vi "Teleop.vi"(10 "Match Info":T1={"Autonomous Elapsed Seconds"=0.0, "TeleOp Elapsed Seconds"=84.436, "Disabled Elapsed Seconds"=0.0, "Visited Autonomous"=FALSE, "Visited TeleOp"=TRUE, "Visited Disabled"=FALSE, "Autonomous Settings"={"Autonomous Style"=enum."Independent", "VI Refnum"=refnum}}, 11 "Call Context":T2=enum."Execute") -> ()   [LabVIEW 2012]
doc: "This VI is called for each TeleOp packet received from the DS where the robot is not disabled. It is often used to read from the joysticks and update I/O or to update setpoints for timed control loops. It should complete and return within 20 milliseconds or it may miss DS packets."
uses:
  <vilib>/Rock Robotics/WPI/DriverStation/WPI_DriverStationDerivedRobotMode.ctl
  <vilib>/Rock Robotics/WPI/DriverStation/WPI_DriverStationMatch Info.ctl
  Controls/Jaguar Control Modes.ctl
  Controls/Robot Orientation.ctl
  Robot Global Data.vi
  Globals/Jaguar Control Mode.vi
  Globals/Autonomous Tipping.vi
  Autonomous/Autonomous Shooting.vi
  Globals/Are We Calibrating Steering.vi
  Globals/DriveSystemMode.vi
  Globals/Max Robot Speed.vi
  Globals/Jaguar Commands.vi
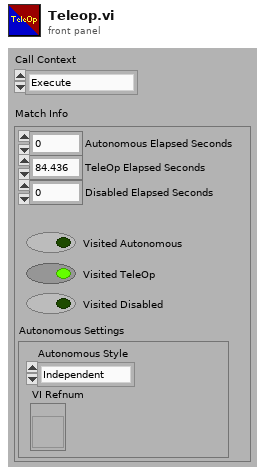
[diagram p1: front panel]
types:
  T1 = typedef "WPI_DriverStationMatch Info.ctl" = cluster{"Autonomous Elapsed Seconds":dbl, "TeleOp Elapsed Seconds":dbl, "Disabled Elapsed Seconds":dbl, "Visited Autonomous":bool, "Visited TeleOp":bool, "Visited Disabled":bool, "Autonomous Settings":cluster{"Autonomous Style":enum16{"Iterative", "Independent"}, "VI Refnum":refnum<vi>}}
  T2 = typedef "WPI_DriverStationDerivedRobotMode.ctl" = enum16{"Init", "Execute", "Stop"}
  T3 = typedef "Jaguar Control Modes.ctl" = enum16{"Speed", "Position"}
  T4 = typedef "Drive System Mode.ctl" = enum16{"Normal", "Crab", "Shoot"}
  T5 = typedef "Robot Orientation.ctl" = enum16{"Landscape", "Portrait"}
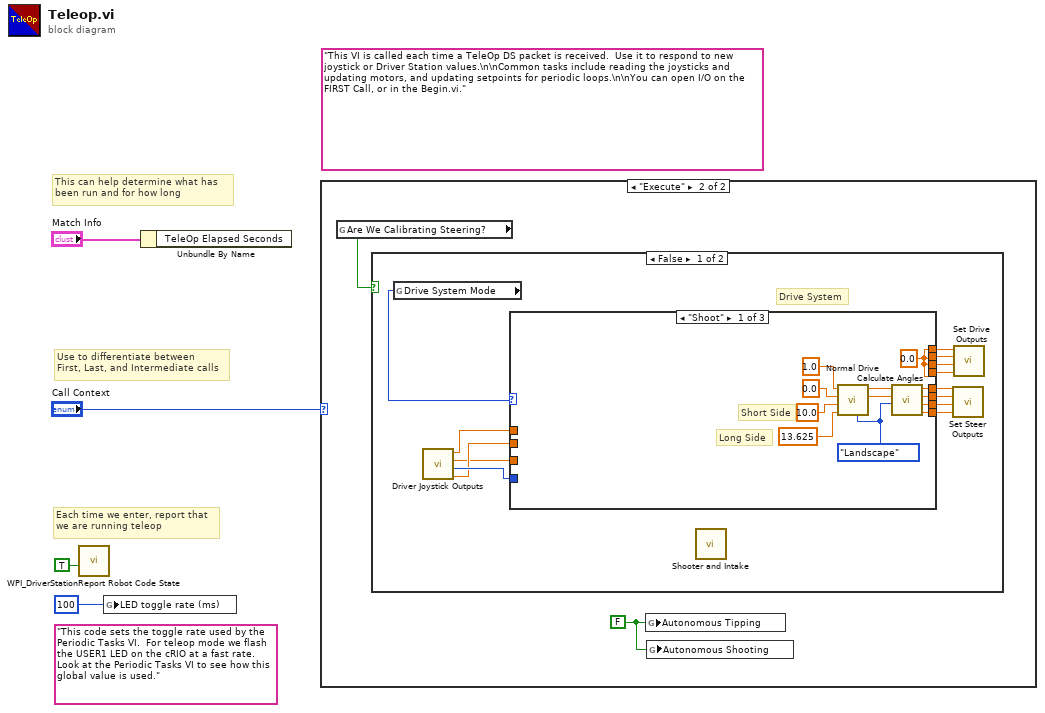
[diagram p0: block diagram]
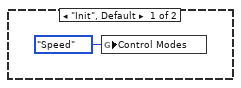
[diagram p2: hidden frame]
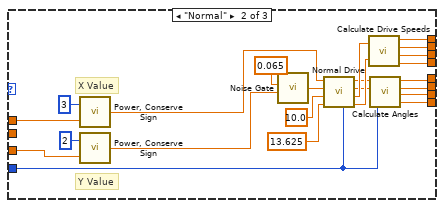
[diagram p3: hidden frame]
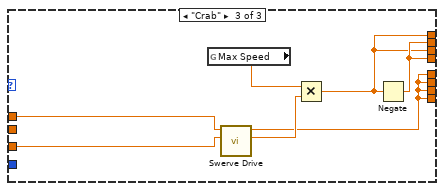
[diagram p4: hidden frame]
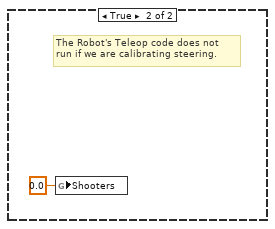
[diagram p5: hidden frame]
diagram:
  (unwired) "This code sets the toggle rate used by the Periodic Tasks VI.  For teleop mode we flash the USER1 LED on the cRIO at a fast rate.  Look at the Periodic Tasks VI to see how this global value is used."
  (unwired) "This VI is called each time a TeleOp DS packet is received.  Use it to respond to new joystick or Driver Station values.\n\nCommon tasks include reading the joysticks and updating motors, and updating setpoints for periodic loops.\n\nYou can open I/O on the FIRST Call, or in the Begin.vi."
  # "Each time we enter, report that\nwe are running teleop"
  # "Use to differentiate between\nFirst, Last, and Intermediate calls"
  # "This can help determine what has\nbeen run and for how long"
  n1 = call <vilib>:"WPI_DriverStationReport Robot Code State.vi"("TeleOp"=TRUE ("Autonomous")) -> ()  [unwired: 10 in, 1 out]
  n2 = global write "Robot Global Data.vi" "LED toggle rate (ms)"(u32 100 ("LED ms toggle rate")) -> ()
  n3 = Unbundle By Name("Match Info") -> ()  [unwired: 1 out]
  n4 = case shown="\"Execute\"" "Call Context" {
    frame "Init", Default {
      n5 = global write "Jaguar Control Mode.vi" "Control Modes"(Jaguar_Control_Modes."Speed" ("Mode")) -> ()
    }
    frame "Execute" {
      w6 = FALSE ("Autonomous Tipping")
      n6 = global read "Are We Calibrating Steering.vi" "Are We Calibrating Steering?"() -> (w7:bool)
      n7 = case shown="False" w7 {
        frame False {
          # "Drive System"
          n8 = global read "DriveSystemMode.vi" "Drive System Mode"() -> (w20:T4)
          n9 = call "Driver Joystick Outputs.vi"() -> ("Joy X"=w8:dbl, "Joy Y"=w9:dbl, "Robot Orientation"=w11:T5, "Joy Twist"=w10:dbl)  [unwired: 3 in]
          n10 = case shown="\"Shoot\"" w20 {
            tunnel: [w28 w47 w60] -> w15
            tunnel: w10 -> [_ _ _]
            tunnel: w9 -> [_ w35 w56]
            tunnel: [w21 w42 w58] -> w19
            tunnel: [w21 w41 w59] -> w18
            tunnel: [w21 w40 w58] -> w17
            tunnel: [w21 w39 w59] -> w16
            tunnel: [w27 w46 w60] -> w14
            tunnel: [w26 w45 w60] -> w13
            tunnel: [w25 w44 w60] -> w12
            tunnel: w11 -> [_ w43 _]
            tunnel: w8 -> [_ w34 w57]
            frame "Shoot" {
              w21 = 0.0 ("Front Left Speed")
              w22 = Robot_Orientation."Landscape" ("Robot Orientation")
              # "Long Side"
              # "Short Side"
              n11 = call "Normal Drive.vi"("Joy X"=1.0, "Joy Y"=0.0, "Short Radius (Inches)"=10.0 ("Vertical Radius (Inches)"), "Long Radius (Inches)"=13.625 ("Lateral Radius (Inches)"), "Robot Orientation"=w22) -> ("Front Left Angle Out"=w24:dbl, "Front Right Angle Out"=w23:dbl)  [unwired: 1 in, 2 out]
              n12 = call "Calculate Angles.vi"("Robot Orientation"=w22, "Right Angle In"=w23, "Left Angle In"=w24) -> ("Rear Right Steer Out"=w25:dbl, "Rear Left Pot Out"=w26:dbl, "Front Right Pot Out"=w27:dbl, "Front Left Pot Out"=w28:dbl)  [unwired: 1 in]
            }
            frame "Normal" {
              # "Y Value"
              # "X Value"
              n13 = call "Power, Conserve Sign.vi"("Input"=w34, "Power"=3) -> ("Output"=w38:dbl)  [unwired: 1 in]
              n14 = call "Power, Conserve Sign.vi"("Input"=w35, "Power"=2) -> ("Output"=w36:dbl)  [unwired: 1 in]
              n15 = call "Noise Gate.vi"("Gate Value"=0.065, "Value In"=w36) -> ("Value Out"=w52:dbl)  [unwired: 5 in]
              n16 = call "Normal Drive.vi"("Joy X"=w38, "Joy Y"=w52, "Short Radius (Inches)"=10.0 ("Vertical Radius (Inches)"), "Long Radius (Inches)"=13.625 ("Lateral Radius (Inches)"), "Robot Orientation"=w43) -> ("Front Left Angle Out"=w49:dbl, "Front Right Angle Out"=w48:dbl, "Left Speed Out"=w51:dbl, "Right Speed Out"=w50:dbl)  [unwired: 1 in]
              n17 = call "Calculate Drive Speeds.vi"("Left Speed In"=w51, "Right Speed In"=w50) -> ("Front Left Speed"=w42:dbl, "Front Right Speed"=w41:dbl, "Rear Left Speed"=w40:dbl, "Rear Right Speed"=w39:dbl)  [unwired: 2 in]
              n18 = call "Calculate Angles.vi"("Robot Orientation"=w43, "Right Angle In"=w48, "Left Angle In"=w49) -> ("Rear Right Steer Out"=w44:dbl, "Rear Left Pot Out"=w45:dbl, "Front Right Pot Out"=w46:dbl, "Front Left Pot Out"=w47:dbl)  [unwired: 1 in]
            }
            frame "Crab" {
              n19 = global read "Max Robot Speed.vi" "Max Speed"() -> (w62:dbl)
              n20 = call "Swerve Drive.vi"("Joy Y"=w56, "Joy X"=w57) -> ("Speed"=w61:dbl, "Wheel Angle"=w60:dbl)  [unwired: 8 in]
              n21 = Multiply(x=w62, y=w61) -> (x*y=w58:dbl)
              n22 = Negate(x=w58) -> (-x=w59:dbl)
            }
          }
          n23 = call "Shooter and Intake.vi"() -> ()  [unwired: 1 in]
          n24 = call "Set Steer Outputs.vi"("Rear Right"=w12, "Rear Left"=w13, "Front Right"=w14, "Front Left"=w15) -> ()  [unwired: 8 in]
          n25 = call "Set Drive Outputs.vi"("Rear Right"=w16, "Rear Left"=w17, "Front Right"=w18, "Front Left"=w19) -> ()  [unwired: 8 in]
        }
        frame True {
          # "The Robot's Teleop code does not \nrun if we are calibrating steering."
          n26 = global write "Jaguar Commands.vi" "Shooters"(0.0 ("Shooters")) -> ()
        }
      }
      n27 = global write "Autonomous Tipping.vi" "Autonomous Tipping"(w6) -> ()
      n28 = global write "Autonomous Shooting.vi" "Autonomous Shooting"(w6) -> ()
    }
  }
